vi "CheckCore.vi"(8 "error in (no error)":errorcluster, 9 "# of Refs":i32, 10 "References":refnum<vi>[](array[refnum]), 11 "Function in":refnum<class "Function.lvclass">) -> (0 "error out":errorcluster, 1 "Reject?":bool, 2 "dup References":refnum<vi>[](array[refnum]), 3 "Function out":refnum<class "Function.lvclass">)   [LabVIEW 2014, in "BuildSecurity.lvlib" / "Function.lvclass"]
doc: "Determines if any blacklisted LabVIEW Function exists in the VI."
uses:
  Function.lvclass
  Blacklist.lvclass/Blacklist.ctl
  ReadItems.vi
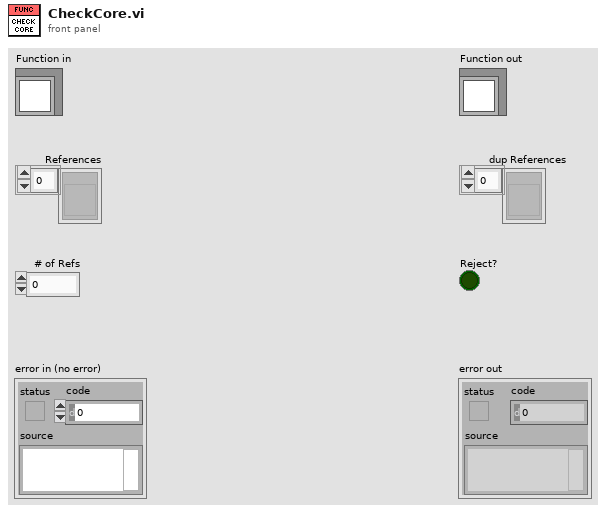
[diagram p1: front panel]
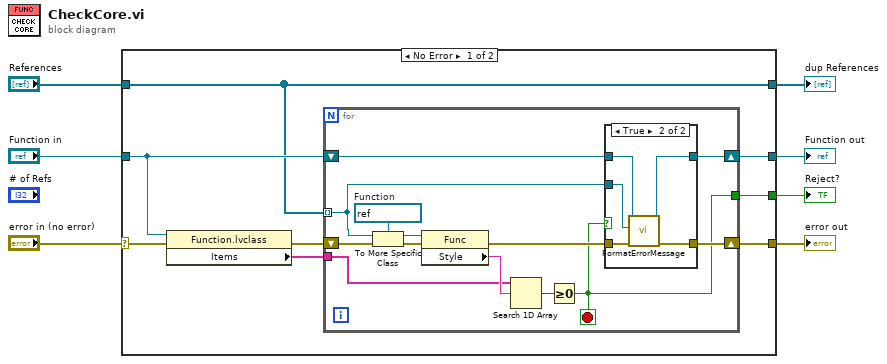
[diagram p0: block diagram]
diagram:
  n1 = case shown="No Error" "error in (no error)" {
    selector: "error in (no error)" -> [w15 w38]
    tunnel: [w10 w38] -> w6
    tunnel: "Function in" -> [w13 w37]
    tunnel: [w9 w37] -> w4
    tunnel: "References" -> [w12 w36]
    tunnel: [w12 w36] -> w2
    tunnel: [w8 _] -> w1
    frame No Error {
      n2 = property class="Function.lvclass"(reference=w13, error in=w15) -> (error out=w11:errorcluster, "Items"=w14:string[])  [unwired: 1 out]
      n3 = for {
        tunnel: w14 -> [w22]
        shift-right: [w19] -> w9
        shift-left: w13 -> [w20]
        tunnel: w12 -> [w17] mode=indexing
        shift-right: [w18] -> w10
        shift-left: w11 -> [w23]
        tunnel: [w16] -> w8
        stop <- w16 stop-if-true
        w28 = refnum<vi> refnum  # Function
        n4 = To More Specific Class(target class=w28, reference=w17, error in=w23) -> (specific class reference=w26:refnum<vi>, error out=w27:errorcluster)
        n5 = property class="Func"(reference=w26, error in=w27) -> (error out=w21:errorcluster, "Style"=w24:string)  [unwired: 1 out]
        n6 = Search 1D Array(1D array=w22, element=w24) -> (index of element=w25:i32)  [unwired: 1 in]
        n7 = Greater Or Equal To 0?(x=w25) -> (x >= 0?=w16:bool)
        n8 = case shown="True" w16 {
          tunnel: w21 -> [w29 w35]
          tunnel: w20 -> [w30 w34]
          tunnel: [w30 w33] -> w19
          tunnel: [w29 w32] -> w18
          tunnel: w17 -> [_ w31]
          frame False {
          }
          frame True {
            n9 = call-dynamic "FormatErrorMessage.vi"("error in (no error)"=w35, "GObj Refnum"=w31, "Blacklist in"=w34) -> ("error out"=w32:errorcluster, "Blacklist out"=w33:refnum<class "Function.lvclass">)  [unwired: 6 in, 1 out]
          }
        }
      }
    }
    frame Error {
    }
  }
  "error out" <- w6
  "Function out" <- w4
  "dup References" <- w2
  "Reject?" <- w1
